vi "add_frames_to_meas_cluster.vi"(3 "meas cluster":T3, 5 "wavefrom array":dbl[][][](array[numeric])) -> (1 "output cluster":T1)   [LabVIEW 2011]
panel:
  in  "frame cluster":T2
  in  "time cluster":T4
  in  "spectra cluster":T5
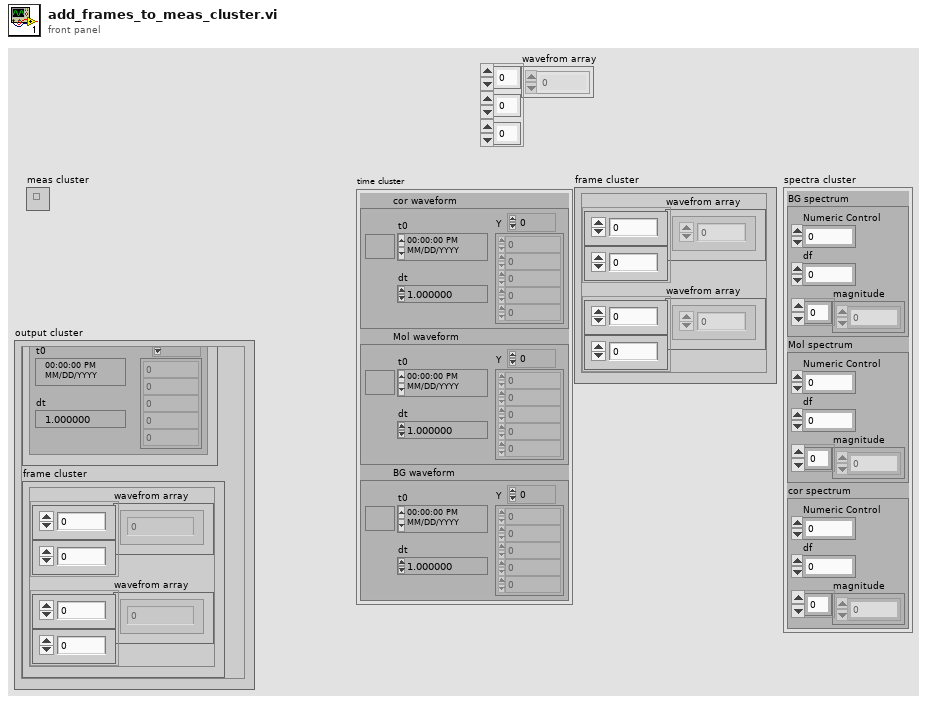
[diagram p1: front panel]
types:
  T1 = cluster{"spectra cluster":cluster{"BG spectrum":cluster{"Numeric Control":dbl, "df":dbl, "magnitude":dbl[]}, "Mol spectrum":cluster{"Numeric Control":dbl, "df":dbl, "magnitude":dbl[]}, "cor spectrum":cluster{"Numeric Control":dbl, "df":dbl, "magnitude":dbl[]}}, "time cluster":cluster{"cor waveform":waveform(dbl), "Mol waveform":waveform(dbl), "BG waveform":waveform(dbl)}, "frame cluster":cluster{"wavefrom array":dbl[][], "wavefrom array":dbl[][]}}
  T2 = cluster{"wavefrom array":dbl[][], "wavefrom array":dbl[][]}
  T3 = cluster{"spectra cluster":cluster{"BG spectrum":cluster{"Numeric Control":dbl, "df":dbl, "magnitude":dbl[]}, "Mol spectrum":cluster{"Numeric Control":dbl, "df":dbl, "magnitude":dbl[]}, "cor spectrum":cluster{"Numeric Control":dbl, "df":dbl, "magnitude":dbl[]}}, "time cluster":cluster{"cor waveform":waveform(dbl), "Mol waveform":waveform(dbl), "BG waveform":waveform(dbl)}}
  T4 = cluster{"cor waveform":waveform(dbl), "Mol waveform":waveform(dbl), "BG waveform":waveform(dbl)}
  T5 = cluster{"BG spectrum":cluster{"Numeric Control":dbl, "df":dbl, "magnitude":dbl[]}, "Mol spectrum":cluster{"Numeric Control":dbl, "df":dbl, "magnitude":dbl[]}, "cor spectrum":cluster{"Numeric Control":dbl, "df":dbl, "magnitude":dbl[]}}
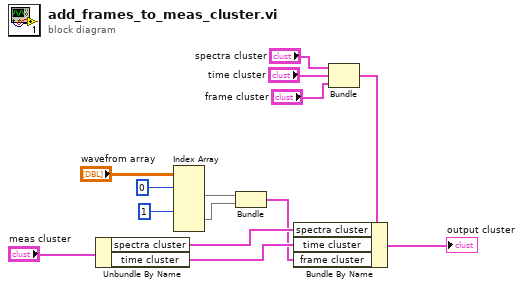
[diagram p0: block diagram]
diagram:
  n1 = Unbundle By Name("meas cluster") -> ("spectra cluster"=w5:T5, "time cluster"=w4:T4)
  n2 = Index Array(array="wavefrom array", index (dim 0) #1=0 ("disabled index (page)"), index (dim 0) #2=1 ("disabled index (page)")) -> (element #1=w7:dbl[][], element #2=w6:dbl[][])  [unwired: 4 in]
  n3 = Bundle("wavefrom array"=w7, "wavefrom array"=w6) -> (w3:T2)  [unwired: 1 in]
  n4 = Bundle("spectra cluster"="spectra cluster", "time cluster"="time cluster", "frame cluster"="frame cluster") -> (w11:T1)  [unwired: 1 in]
  n5 = Bundle By Name(cluster=w11, "spectra cluster"=w5, "time cluster"=w4, "frame cluster"=w3) -> (→"output cluster":T1)
